vi "Create Guardian Personal Log.vi"(8 "error in (no error)":errorcluster, 11 "Guardian in":refnum<class "Guardian.lvclass">) -> (0 "error out":errorcluster, 3 "Guardian out":refnum<class "Guardian.lvclass">)   [LabVIEW 2026, in "TALOS.lvlib" / "Guardian.lvlib" / "Guardian.lvclass"]
uses:
  Guardian.lvclass
  Ancestor/Ancestor/Ancestor.lvclass/Ancestor.ctl
  Guardian.lvclass/Guardian.ctl
  Support VIs/Generate Error.vi
  FGV/Error Memory/Get Error Description.vi
  Support VIs/Get PC name.vi
  Ancestor/Ancestor/Read ID.vi
  Support VIs/Get Class Name.vi
  <vilib>/Utility/error.llb/Clear Errors.vi
  FGV/Error Memory/Error Memory Core.vi
  <vilib>/AdvancedString/Delimited String to 1D String Array.vi
  <vilib>/AdvancedString/Delimited String to 1D String Array (string).vi
  Support VIs/Circus Root Path.vi
  FGV/Error Memory/Error Crt Lvl checker.vi
  FGV/Error Memory/Error Memory Core.vi/40c8088d-b597-4017-91af-faa98e00292e.vi
  FGV/Error Memory/Error Memory Core.vi/d4a3ab98-063c-4e44-b43d-fbdcfe6c2be2.vi
  Support VIs/Global Memory.vi
  <vilib>/Utility/LVClass/Get LV Class Name.vi
  Support VIs/Is in Packed Library.vi
  Support VIs/TALOS Root path.vi
  Support VIs/Read CSV worksheet.vi
  Support VIs/Global Constants.vi
  <vilib>/Utility/error.llb/General Error Handler.vi
  <vilib>/Utility/config.llb/Open Config Data.vi
  <vilib>/Utility/config.llb/Get Section Names.vi
  <vilib>/Utility/config.llb/Get Key Names.vi
  <vilib>/Utility/config.llb/Read Key.vi
  <vilib>/Utility/config.llb/Read Key (String).vi
  <vilib>/Utility/config.llb/Close Config Data.vi
  Ancestor/Ancestor/Ancestor.lvclass
  <vilib>/Comparison/Equal/Equal Functor/Equal Functor.lvclass
  Classes/Log/Log.lvclass
  TALOS.lvlib
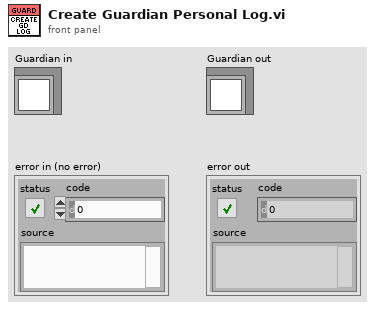
[diagram p1: front panel]
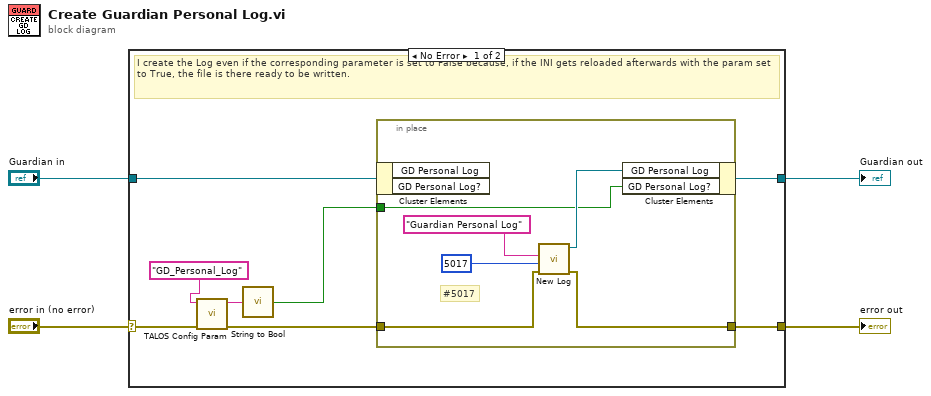
[diagram p0: block diagram]
diagram:
  n1 = case shown="No Error" "error in (no error)" {
    selector: "error in (no error)" -> [w9 w19]
    tunnel: [w12 w19] -> w4
    tunnel: "Guardian in" -> [w11 w20]
    tunnel: [w10 w20] -> w1
    frame No Error {
      # "I create the Log even if the corresponding parameter is set to False because, if the INI gets reloaded afterwards with the param set to True, the file is there ready to be written."
      n2 = call "TALOS Config Param.vi"("error in (no error)"=w9, "Parameter Name"="GD_Personal_Log") -> ("error out"=w8:errorcluster, "Output"=w6:string)  [unwired: 8 in]
      n3 = call "String to Bool.vi"("String"=w6) -> ("Boolean"=w5:bool)
      n4 = in-place {
        in-place-border: w8 -> [w16]
        in-place-border: [w17] -> w12
        in-place-border: w5 -> [w13]
        # "#5017"
        n5 = in-place-cluster #1(w11) -> ()  [unwired: 2 out]
        n6 = call "New Log.vi"("error in (no error)"=w16, "Specific Error Code"=5017, "Name"="Guardian Personal Log") -> ("error out"=w17:errorcluster, "Log out"=w18:refnum<class "Log.lvclass">)  [unwired: 7 in]
        n7 = in-place-cluster #1("GD Personal Log"=w18, "GD Personal Log?"=w13) -> (w10:refnum<class "Guardian.lvclass">)
      }
    }
    frame Error {
    }
  }
  "error out" <- w4
  "Guardian out" <- w1
